vi "Create.vi"(7 "Direction":T1, 8 "error in (no error)":errorcluster, 9 "Custom Config Data":u8[](array[numeric]), 10 "Name":string, 11 "CIF_Fifo_U8 in":refnum<class "CIF_Fifo_L2Enet_Multi.lvclass">) -> (0 "error out":errorcluster, 3 "CIF_Fifo_U8 out":refnum<class "CIF_Fifo_L2Enet_Multi.lvclass">)   [LabVIEW 2021, in "CIF_Fifo_L2Enet_Multi.lvclass"]
uses:
  CIF_Fifo_L2Enet_Multi.lvclass
  D:/dev/Packages/Channel_Manager/src/CIFChannels/CIFChannels.lvclass
  D:/dev/Packages/Channel_Manager/src/CIF_NIChn/NIChn/CIF_NIChn.lvclass
  D:/dev/Packages/Channel_Manager/src/CIF_NIChn/FIFO_U8/CIF_NIChn_Fifo_U8.lvclass
  CIFChannels/Typedef/Direction.ctl
  CIFChannels/Typedef/Disconnect Behavior.ctl
  CIFChannels/CIFChannels.lvclass/CIFChannels.ctl
  <vilib>/CIF Foundation/CIF Utilities/Statistics/I64/Stats_I64_CIF_U.lvclass/Stats_I64_CIF_U.ctl
  CIFChannels/Typedef/Channel State.ctl
  NIChn/CIF_NIChn.lvclass/CIF_NIChn.ctl
  FIFO_U8/CIF_NIChn_Fifo_U8.lvclass/CIF_NIChn_Fifo_U8.ctl
  6cf79c70-debc-41de-b122-58e2a501a1fe.vi
  CIFChannels/Accessors/Write Channel State.vi
  NIChn/Accessors/Write CIF Channel.vi
  CIFChannels/Accessors/Write Channel Benchmark.vi
  CIFChannels/Accessors/Write Flatten Benchmark.vi
  FIFO_U8/Accessors/Write Payload.vi
  CIFChannels/SubVIs/Get Type from Class.vi
  ChannelCommon/Utilities/Unflatten FIFO Config.vi
  CIFChannels/Utilities/Apply Flags.vi
  CIFChannels/Accessors/Write Type.vi
  CIFChannels/Accessors/Write Channel Class.vi
  CIFChannels/Accessors/Write Direction.vi
  CIFChannels/Accessors/Write Tag Disconnect Behavior.vi
  CIFChannels/Accessors/Write Name.vi
  CIFChannels/Accessors/Write Custom Config Data.vi
  <vilib>/CIF Foundation/CIF Channels/CIFChannels/SubVIs/Add Error.vi
  6cf79c70-debc-41de-b122-58e2a501a1fe.vi/c28b0ead-42ad-4072-80a2-aca7f2bd7ce3.vi
  <vilib>/CIF Foundation/CIF Channels/CIFChannels/SubVIs/CIFServices Fill In Error Info Ex.vi
  <vilib>/CIF Foundation/CIF Channels/CIFChannels/SubVIs/Get dll Path.vi
  <vilib>/CIF Foundation/CIF Utilities/DataTypes/Unflatten U64.vi
  ChannelCommon/Utilities/Expand FIFO Flags.vi
  <vilib>/CIF Foundation/CIF Utilities/Errors/Append Error Location.vi
  <vilib>/Utility/LVClass/Get LV Class Name.vi
  <vilib>/CIF Foundation/CIF Utilities/Statistics/I64/Stats_I64_CIF_U.lvclass
  CIFChannels/CIFChannels.lvclass
  ChannelCommon/ChannelCommon.lvlib
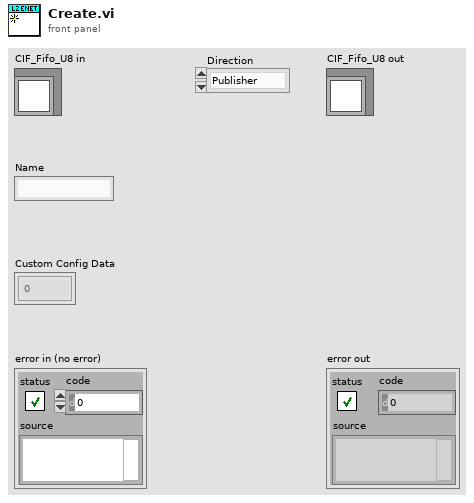
[diagram p1: front panel]
types:
  T1 = typedef "CIFChannels.lvclass/Direction.ctl" = enum16{"Publisher", "Subscriber"}
  T2 = typedef "CIFChannels.lvclass/Disconnect Behavior.ctl" = enum16{"Default value", "Last value", "Error with default"}
  T3 = typedef "CIFChannels.lvclass/Channel State.ctl" = enum16{"Creating", "Disconnected", "Connecting", "Connected", "Destroyed"}
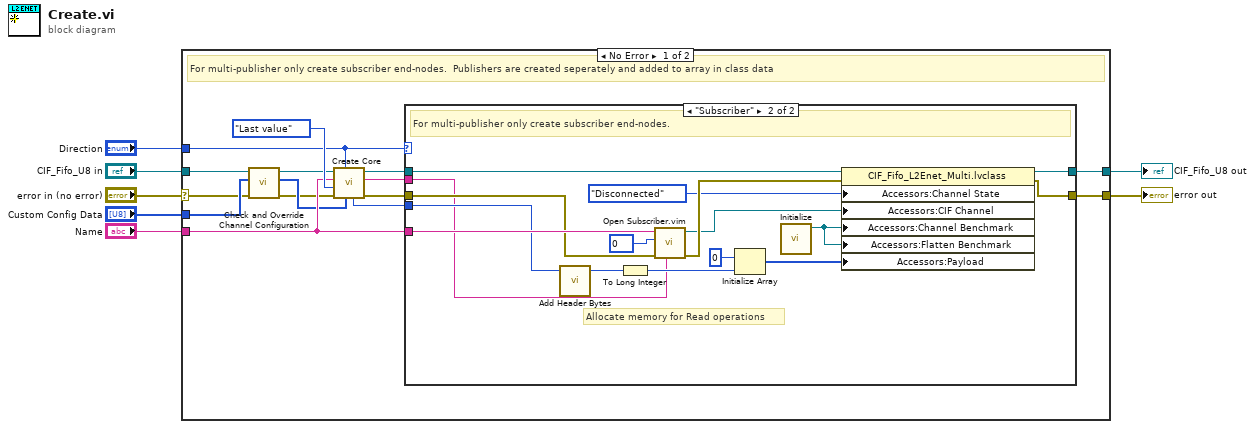
[diagram p0: block diagram]
diagram:
  n1 = case shown="No Error" "error in (no error)" {
    selector: "error in (no error)" -> [w16 w42]
    tunnel: [w10 w42] -> w2
    tunnel: [w11 w41] -> w1
    tunnel: "CIF_Fifo_U8 in" -> [w19 w41]
    tunnel: "Name" -> [w21 _]
    tunnel: "Direction" -> [w13 _]
    tunnel: "Custom Config Data" -> [w18 _]
    frame No Error {
      # "For multi-publisher only create subscriber end-nodes.  Publishers are created seperately and added to array in class data"
      n2 = call-dynamic "Check and Override Channel Configuration.vi"("error in (no error)"=w16, "Custom Config Data in"=w18, "CIF_Fifo_L2Enet_Multi in"=w19) -> ("error out"=w15:errorcluster, "Custom Config Data out"=w17:u8[], "CIF_Fifo_L2Enet_Multi out"=w14:refnum<class "CIF_Fifo_L2Enet_Multi.lvclass">)  [unwired: 6 in]
      n3 = call "Create Core.vi"("Custom Config Data"=w17, "Direction"=w13, "error in (no error)"=w15, "Disconnect Behavior"=Disconnect_Behavior."Last value", "Name"=w21, "CIFChannels in"=w14) -> ("error out"=w20:errorcluster, "Channel Type"=w8:string, "CIFChannels out"=w12:refnum<class "CIF_Fifo_L2Enet_Multi.lvclass">, "Bytes/Msg"=w9:u64)  [unwired: 1 in, 1 out]
      n4 = case shown="\"Subscriber\"" w13 {
        tunnel: w21 -> [_ w40]
        tunnel: w20 -> [w24 w39]
        tunnel: w12 -> [w23 w34]
        tunnel: [w23 w29] -> w11
        tunnel: [w24 w28] -> w10
        tunnel: w9 -> [_ w27]
        tunnel: w8 -> [_ w25]
        frame "Publisher", Default {
          # "Publishers are created seperately and added to array in class data"
        }
        frame "Subscriber" {
          # "Allocate memory for Read operations"
          # "For multi-publisher only create subscriber end-nodes."
          n5 = call "Add Header Bytes.vi"("Bytes/Msg"=w27) -> ("Bytes/Msg with header"=w26:u64)  [unwired: 3 in]
          n6 = To Long Integer(number=w26) -> (32bit integer=w38:i32)
          n7 = call "Open Subscriber.vim"("Channel Type Description"=w25, "error in"=w39, "Input Type"=u8 0, "Channel Name"=w40) -> ("error out"=w33:errorcluster, "CIF Channel"=w31:refnum<k21>)  [unwired: 6 in]
          n8 = Initialize Array(u8 0 ("Numeric"), w38) -> (w30:u8[])
          n9 = call <vilib>:"Initialize.vi"() -> ("Stats_I64_CIF_U out"=w35:refnum<class "Stats_I64_CIF_U.lvclass">)  [unwired: 10 in, 1 out]
          n10 = property class="CIF_Fifo_L2Enet_Multi.lvclass"(reference=w34, error in=w33, "Accessors:Channel State"=Channel_State."Disconnected" ("Channel State"), "Accessors:CIF Channel"=w31, "Accessors:Channel Benchmark"=w35, "Accessors:Flatten Benchmark"=w35, "Accessors:Payload"=w30) -> (reference out=w29:refnum<class "CIF_Fifo_L2Enet_Multi.lvclass">, error out=w28:errorcluster)
        }
      }
    }
    frame Error {
    }
  }
  "error out" <- w2
  "CIF_Fifo_U8 out" <- w1
